vi "SerialInToQueue.vi"(8 "error in (no error)":errorcluster, 10 "VISA resource name in":refnum<visa-resource-name>, 11 "Queue in":refnum<queue>) -> (0 "error out":errorcluster, 1 "VISA resource name":refnum<visa-resource-name>, 2 "read buffer":string, 3 "Queue out":refnum<queue>)   [LabVIEW 2013]
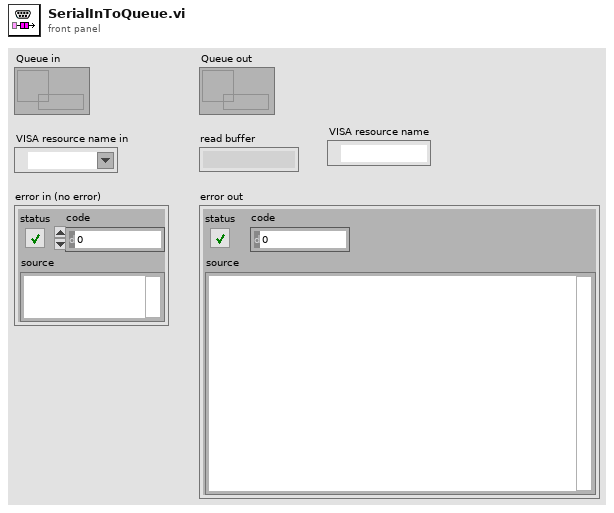
[diagram p1: front panel]
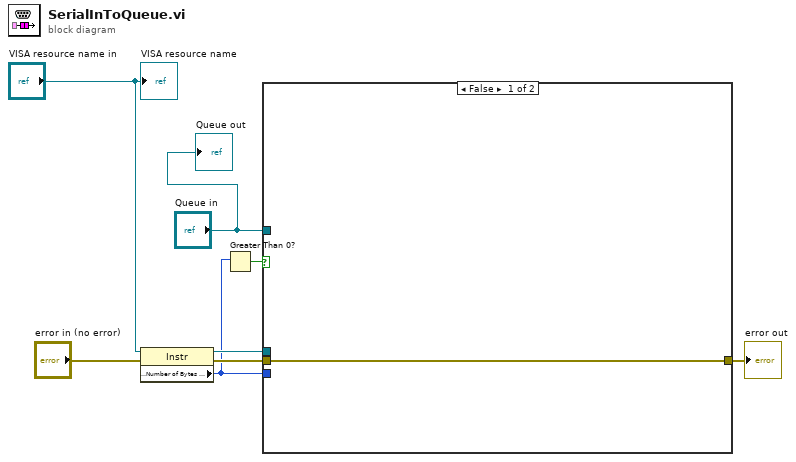
[diagram p0: block diagram]
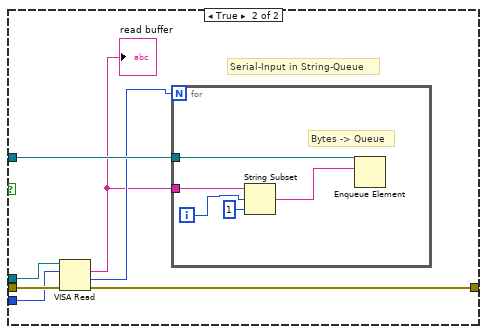
[diagram p2: hidden frame]
diagram:
  n1 = property class="Instr"(reference="VISA resource name in", error in="error in (no error)") -> (reference out=w5:refnum<visa-resource-name>, error out=w6:errorcluster, "Serial Settings:Number of Bytes at Serial Port"=w3:u32)
  n2 = Greater Than 0?(x=w3) -> (x > 0?=w4:bool)
  n3 = case shown="False" w4 {
    tunnel: w6 -> [w9 w16]
    tunnel: w5 -> [_ w15]
    tunnel: w3 -> [_ w14]
    tunnel: [w9 w13] -> w2
    tunnel: "Queue in" -> [_ w12]
    frame False {
    }
    frame True {
      # "Serial-Input in String-Queue"
      n4 = VISA Read(VISA resource name=w15, byte count=w14, error in (no error)=w16) -> (read buffer=w10:string, return count=w11:u32, error out=w13:errorcluster)  [unwired: 1 out]
      "read buffer" <- w10
      n5 = for {
        N: w11 -> [_]
        tunnel: w12 -> [w21]
        tunnel: w10 -> [w20]
        i -> [w18]
        # "Bytes -> Queue"
        n6 = String Subset(string=w20, offset (0)=w18, length (rest)=1 ("length (rest)")) -> (substring=w17:string)
        n7 = Enqueue Element(queue=w21, element=w17) -> ()  [unwired: 2 in, 3 out]
      }
    }
  }
  "error out" <- w2
  "VISA resource name" <- "VISA resource name in"
  "Queue out" <- "Queue in"
